vi "2d_array_from_ini.vi"(11 "Ini gene W":string) -> (3 "Array":dbl[][](array[numeric]))   [LabVIEW 2018]
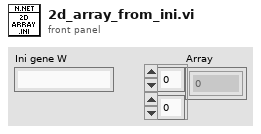
[diagram p1: front panel]
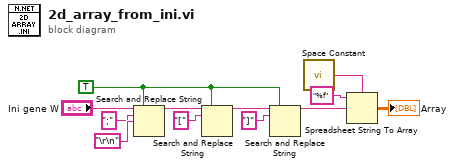
[diagram p0: block diagram]
diagram:
  w12 = TRUE ("replace all? (F)")
  n1 = Search and Replace String(replace all?=w12, input string="Ini gene W", search string=";" ("format string"), replace string="\r\n") -> (result string=w7:string)  [unwired: 4 in, 3 out]
  n2 = Search and Replace String(replace all?=w12, input string=w7, search string="[" ("input string")) -> (result string=w8:string)  [unwired: 5 in, 3 out]
  n3 = Search and Replace String(replace all?=w12, input string=w8, search string="]") -> (result string=w10:string)  [unwired: 5 in, 3 out]
  n4 = call <vilib>:"Space Constant.vi"() -> ("String"=w3:string)
  n5 = Spreadsheet String To Array(delimiter (Tab)=w3, format string="%f", spreadsheet string=w10) -> (array=→"Array":dbl[][])  [unwired: 1 in]
